vi "Try Get Sub Object.vi"(8 "error in":errorcluster, 9 "Sub Index":u8 format="%02x", 10 "Index":u16 format="%04x", 11 "Object Dictionary in":refnum<class "Object Dictionary.lvclass">) -> (0 "error out":errorcluster, 1 "Sub Object":refnum<class "Sub Object.lvclass">, 2 "Success":bool, 3 "Object Dictionary out":refnum<class "Object Dictionary.lvclass">)   [LabVIEW 2020, in "CANopen.lvlib" / "Object Dictionary.lvclass"]
doc: "When this method returns, contains the value associated with the specified key, if the key is found; otherwise, the default value for the type of the value parameter. This parameter is passed uninitialized."
uses:
  Object Dictionary.lvclass
  Sub Object/Sub Object.lvclass
  Object Dictionary.lvclass/Object Dictionary.ctl
  Object Entry/Object Entry.lvclass
  Ordered-Dictionary/Ordered Object Dictionary/Source/Ordered Object Dictionary.lvclass
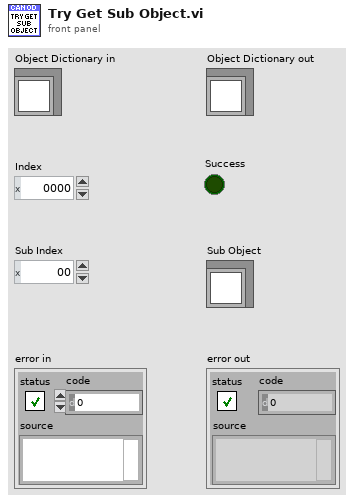
[diagram p1: front panel]
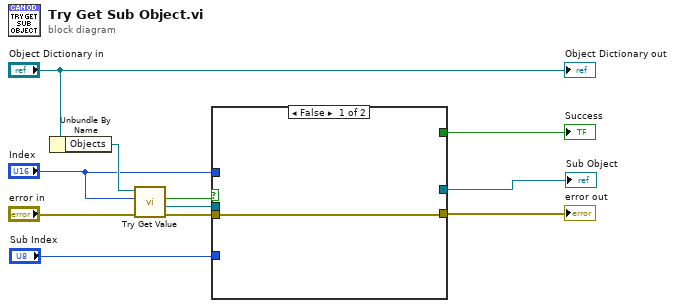
[diagram p0: block diagram]
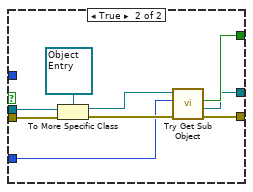
[diagram p2: hidden frame]
diagram:
  n1 = Unbundle By Name("Object Dictionary in") -> ("Objects"=w8:refnum<class "Ordered Object Dictionary.lvclass">)
  n2 = call "Try Get Value.vi"("error in"="error in", "Key"="Index", "Ordered Object Dictionary in"=w8) -> ("error out"=w11:errorcluster, "Value"=w7:refnum<class>, "Success"=w6:bool)  [unwired: 5 in, 1 out]
  n3 = case shown="False" w6 {
    tunnel: w11 -> [w12 w21]
    tunnel: w7 -> [_ w20]
    tunnel: [_ w13] -> w2
    tunnel: "Index" -> [_ _]
    tunnel: "Sub Index" -> [_ w17]
    tunnel: [w12 w15] -> w3
    tunnel: [_ w14] -> w1
    frame False {
    }
    frame True {
      n4 = To More Specific Class(target class=refnum<class "Object Entry.lvclass"> refnum ("CANopen.lvlib:Obj Entry"), reference=w20, error in=w21) -> (specific class reference=w16:refnum<class "Object Entry.lvclass">, error out=w18:errorcluster)
      n5 = call "Try Get Sub Object.vi"("error in"=w18, "Sub Index"=w17, "Obj Entry in"=w16) -> ("error out"=w15:errorcluster, "Sub Object"=w13:refnum<class "Sub Object.lvclass">, "Success"=w14:bool)  [unwired: 5 in, 1 out]
    }
  }
  "error out" <- w3
  "Success" <- w1
  "Sub Object" <- w2
  "Object Dictionary out" <- "Object Dictionary in"
